vi "SubVI RX Test.vi"(7 "number of samples":i64=-1, 8 "error in (no error)":errorcluster, 9 "reference position":dbl format="%0.2f", 10 "trigger level":dbl format="%0.2f", 11 "session handle":refnum<k15>) -> (0 "error out":errorcluster, 1 "packet found":bool, 2 "IQ Waveform":cluster{"t0":dbl, "dt":dbl, "Y":cdb[]}, 3 "session handle out":refnum<k15>)   [LabVIEW 2015]
uses:
  <instrlib>/niUSRP/niUSRP Fetch Rx Data (CDB Cluster).vi
  <vilib>/Analysis/NI_AALPro.lvlib
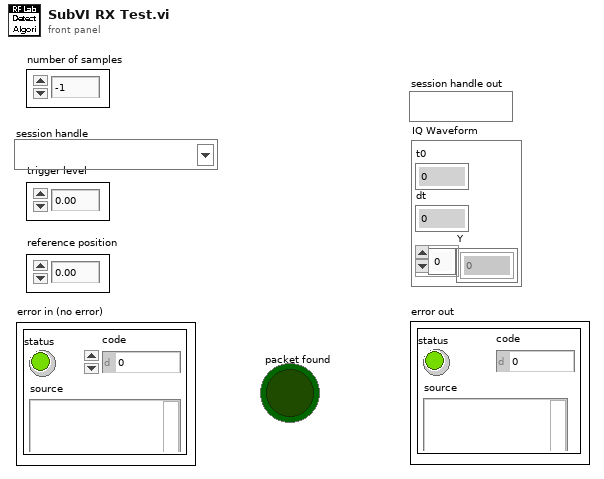
[diagram p1: front panel]
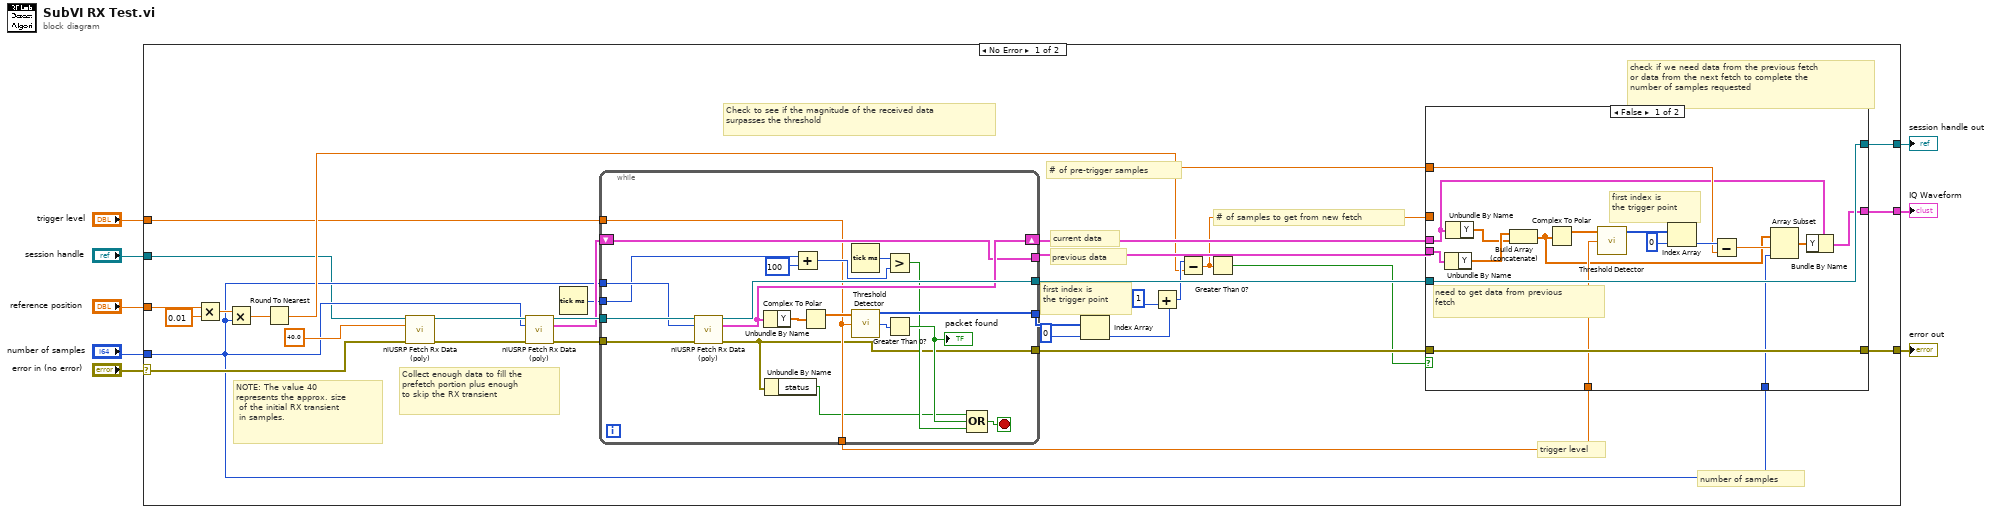
[diagram p0: block diagram]
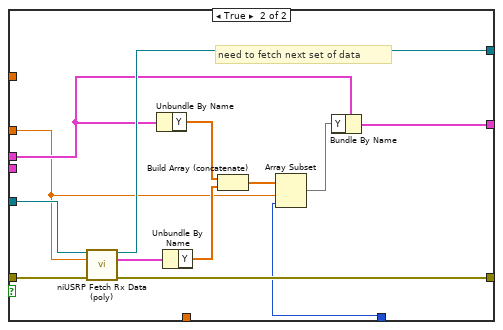
[diagram p2: hidden frame]
diagram:
  n1 = case shown="No Error" "error in (no error)" {
    selector: "error in (no error)" -> [w18 w90]
    tunnel: [w21 w90] -> w8
    tunnel: "number of samples" -> [w14 _]
    tunnel: "reference position" -> [w13 _]
    tunnel: "session handle" -> [w12 _]
    tunnel: "trigger level" -> [w11 _]
    tunnel: [w10 _] -> w2
    tunnel: [w9 _] -> w1
    frame No Error {
      # "trigger level"
      # "check if we need data from the previous fetch\nor data from the next fetch to complete the \nnumber of samples requested"
      # "number of samples"
      # "# of pre-trigger samples"
      # "current data"
      # "previous data"
      # "NOTE: The value 40\nrepresents the approx. size\n of the initial RX transient\n in samples."
      # "Collect enough data to fill the\nprefetch portion plus enough\nto skip the RX transient"
      # "# of samples to get from new fetch"
      # "first index is \nthe trigger point"
      # "Check to see if the magnitude of the received data\nsurpasses the threshold"
      n2 = Multiply(x=w13, y=0.01) -> (x*y=w38:dbl)
      n3 = Multiply(x=w38, y=w14) -> (x*y=w37:dbl)
      n4 = Round To Nearest(number=w37) -> (nearest integer value=w15:dbl)
      n5 = call-poly <instrlib>:"niUSRP Fetch Rx Data (poly).vi"("session handle"=w12, "number of samples"=40.0 ("x"), "error in (no error)"=w18) -> ("session handle out"=w20:refnum<k15>, "error out"=w19:errorcluster)  [unwired: 9 in, 2 out]
      n6 = call-poly <instrlib>:"niUSRP Fetch Rx Data (poly).vi"("session handle"=w20, "number of samples"=w14, "error in (no error)"=w19) -> ("session handle out"=w25:refnum<k15>, "data"=w23:cluster{"t0":dbl, "dt":dbl, "Y":cdb[]}, "error out"=w24:errorcluster)  [unwired: 9 in, 1 out]
      n7 = Tick Count (ms)() -> (millisecond timer value=w22:u32)
      n8 = while {
        tunnel: [w89] -> w32
        tunnel: [w71] -> w31
        tunnel: [w87] -> w36
        shift-right: [w86] -> w33
        shift-left: w23 -> [w85]
        tunnel: [w85] -> w34
        tunnel: w25 -> [w84]
        tunnel: w14 -> [w83]
        tunnel: w24 -> [w82]
        tunnel: w11 -> [w72]
        tunnel: w22 -> [w78]
        tunnel: [w72] -> w16
        stop <- w79 stop-if-true
        n9 = call-poly <instrlib>:"niUSRP Fetch Rx Data (poly).vi"("session handle"=w84, "number of samples"=w83, "error in (no error)"=w82) -> ("session handle out"=w89:refnum<k15>, "data"=w86:cluster{"t0":dbl, "dt":dbl, "Y":cdb[]}, "error out"=w71:errorcluster)  [unwired: 9 in, 1 out]
        n10 = Unbundle By Name(w86) -> ("Y"=w81:cdb[])
        n11 = Unbundle By Name(w71) -> ("status"=w70:bool)
        n12 = Add(x=w78, y=u32 100) -> (x+y=w75:u32)
        n13 = Complex To Polar(r * e^(i*theta)=w81) -> (r=w80:dbl[])  [unwired: 1 out]
        n14 = Tick Count (ms)() -> (millisecond timer value=w76:u32)
        n15 = call <vilib>:"Threshold Detector.vi"("threshold"=w72, "X"=w80) -> ("count"=w88:i32, "Indices"=w87:i32[])  [unwired: 1 in, 1 out]
        n16 = Greater?(x=w76, y=w75) -> (0:w73:bool)
        n17 = Greater Than 0?(x=w88) -> (x > 0?=w74:bool)
        "packet found" <- w74
        n18 = Compound Arithmetic op=OR(w70, w74, w73) -> (w79:bool)
      }
      n19 = Index Array(array=w36, index=0) -> (element=w28:i32)
      n20 = Add(x=w28, y=1) -> (x+y=w26:i32)
      n21 = Subtract(x=w26, y=w15) -> (x-y=w29:dbl)
      n22 = Greater Than 0?(x=w29) -> (x > 0?=w30:bool)
      n23 = case shown="False" w30 {
        tunnel: w34 -> [w54 _]
        tunnel: w33 -> [w41 w65]
        tunnel: w32 -> [w55 w69]
        tunnel: w31 -> [w56 w68]
        tunnel: w29 -> [_ w59]
        tunnel: [w55 w67] -> w10
        tunnel: [w56 w66] -> w21
        tunnel: [w40 w64] -> w9
        tunnel: w14 -> [w43 w58]
        tunnel: w16 -> [w50 _]
        tunnel: w15 -> [w46 _]
        frame False {
          # "first index is \nthe trigger point"
          # "need to get data from previous\nfetch"
          n24 = Unbundle By Name(w54) -> ("Y"=w53:cdb[])
          n25 = Unbundle By Name(w41) -> ("Y"=w52:cdb[])
          n26 = Build Array (concatenate)(w53, w52) -> (w44:cdb[])
          n27 = Complex To Polar(r * e^(i*theta)=w44) -> (r=w51:dbl[])  [unwired: 1 out]
          n28 = call <vilib>:"Threshold Detector.vi"("threshold"=w50, "X"=w51) -> ("Indices"=w48:i32[])  [unwired: 1 in, 2 out]
          n29 = Index Array(array=w48, index=0) -> (element=w47:i32)
          n30 = Subtract(x=w47, y=w46) -> (x-y=w45:dbl)
          n31 = Array Subset(array=w44, index=w45, length=w43) -> (w42:cdb[])
          n32 = Bundle By Name(cluster=w41, "Y"=w42) -> (w40:cluster{"t0":dbl, "dt":dbl, "Y":cdb[]})
        }
        frame True {
          # "need to fetch next set of data"
          n33 = call-poly <instrlib>:"niUSRP Fetch Rx Data (poly).vi"("session handle"=w69, "number of samples"=w59, "error in (no error)"=w68) -> ("session handle out"=w67:refnum<k15>, "data"=w63:cluster{"t0":dbl, "dt":dbl, "Y":cdb[]}, "error out"=w66:errorcluster)  [unwired: 9 in, 1 out]
          n34 = Unbundle By Name(w65) -> ("Y"=w62:cdb[])
          n35 = Unbundle By Name(w63) -> ("Y"=w61:cdb[])
          n36 = Build Array (concatenate)(w62, w61) -> (w60:cdb[])
          n37 = Array Subset(array=w60, index=w59, length=w58) -> (w57:cdb[])
          n38 = Bundle By Name(cluster=w65, "Y"=w57) -> (w64:cluster{"t0":dbl, "dt":dbl, "Y":cdb[]})
        }
      }
    }
    frame Error {
    }
  }
  "error out" <- w8
  "session handle out" <- w2
  "IQ Waveform" <- w1
